vi "niRFUtil TRC Trace to Waveform (complex wfm).vi"(7 "Measurement Trace":T1 format="%.2f") -> (8 "Complex Waveform":T2 {"y" format="%.2f"; "dx" format="%^.2e"; "x0" format="%^.2e"})   [LabVIEW 2015, in "niRFUtil.lvlib"]
doc: "(c) Copyright 2006, National Instruments, Inc. This VI may not be duplicated, sold, or distributed without written consent from National Instruments."
uses:
  niRFUtil.lvlib
  Includes/niRFUtil INC Complex Waveform.ctl
  Includes/niRFUtil INC Complex Array.ctl
  Includes/niRFUtil INC Trace.ctl
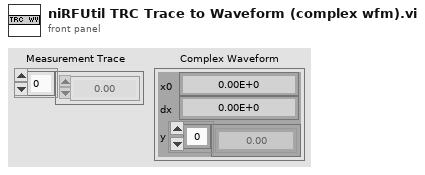
[diagram p1: front panel]
types:
  T1 = typedef "niRFUtil.lvlib/niRFUtil INC Trace.ctl" = sgl[]
  T2 = typedef "niRFUtil.lvlib/niRFUtil INC Complex Waveform.ctl" = cluster{"x0":dbl, "dx":dbl, "y":T3}
  T3 = typedef "niRFUtil.lvlib/niRFUtil INC Complex Array.ctl" = csg[]
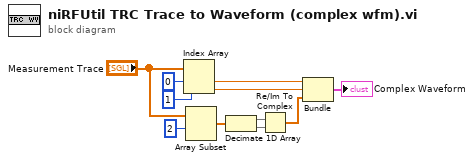
[diagram p0: block diagram]
diagram:
  n1 = Index Array(array="Measurement Trace", index #1=0 ("index"), index #2=1 ("index")) -> (element #1=w3:sgl, element #2=w2:sgl)
  n2 = Array Subset(array="Measurement Trace", index=2) -> (w1:T1)  [unwired: 1 in]
  n3 = Decimate 1D Array(w1) -> (w11:sgl[], w10:sgl[])
  n4 = Re/Im To Complex(1:w10, 2:w11) -> (0:w9:csg[])
  n5 = Bundle("Numeric"=w3, "Numeric"=w2, w9) -> (→"Complex Waveform":cluster{"Numeric":sgl, "Numeric":sgl, csg[]})  [unwired: 1 out]
